vi "Process_Setting_UI2.vi"(9 "Image In":T2, 10 "PreProcess":T1=enum."G_Threshold", 11 "DataIn":string) -> (1 "ExitFLG":bool=TRUE, 3 "DataOut":string)   [LabVIEW 2019]
uses:
  Controls/MaskParam_Type.ctl
  Controls/ParticleFilterParam_Type.ctl
  Controls/LookupTableParam.ctl
  Controls/FiltersParam_Type.ctl
  Controls/GrayMorphologyParam_Type.ctl
  Controls/OperatorsParam_Type.ctl
  Controls/BinaryMonoParam_Type.ctl
  Controls/ExtractPlanParam_Type.ctl
  Controls/UI_Process_Type.ctl
  Controls/ProcessBrightness.ctl
  <vilib>/vision/Image Controls.llb/IMAQ Image.ctl
  Ctrl/VisionProcessName.ctl
  Controls/ProcessColorThreshold.ctl
  Controls/Process_Setting.ctl
  30020945-ae28-4489-8016-9b1403305c34.vi
  ebb7c46e-89fc-4514-88ba-51094c50cf0f.vi
  e91a7cad-c41a-4cff-b925-06470bbe3936.vi
  b75ec72d-941b-4609-8ea7-277ce8708de0.vi
  47af210a-8923-444f-9ea8-79f9655d5eab.vi
  a8380952-e245-4862-98bc-7050634aa2b9.vi
  c91c66e3-d08b-4d8f-9520-13536894a5b1.vi
  b6b5b608-5e76-4822-9d65-04a57b09488a.vi
  97fa0709-478f-42d9-9b21-5a1c8d8fbb1e.vi
  9fa7adbb-d216-4a6e-bf6a-ec4f0884b3b2.vi
  99202b2e-11d4-433c-aa93-4f5d47ce0152.vi
  de4bf947-11f1-4644-b15e-f20b2debb1f4.vi
  d1f0ac64-7591-4813-b16e-cc2f2336aeb7.vi
  21e68b17-46f9-4e60-a793-2575703a9335.vi
  2b11d1c0-0739-46ad-be8a-3e73a10ae897.vi
  6a6545d9-b3d5-4342-817e-e9b56ae9a0c9.vi
  33d971b2-c2c9-4da8-8c72-03e55e502448.vi
  e97b490d-7b27-4472-b442-b6ae32428c3c.vi
  <vilib>/JDP Science/JSONtext/Variant to JSON Text.vi
  <vilib>/JDP Science/JSONtext/JSON text to Variant.vi
  ccb8fe9b-0148-4a2a-9ee9-959eed898db8.vi
  76e84c50-6107-4eeb-8902-48fd924c973a.vi
  068fea54-6e28-4c40-a19e-0b6ebeaa2479.vi
  293cadd9-7c19-42b2-90f6-8eb66fc12dc6.vi
  ad7b33dd-2a70-464f-aced-769d5ac39227.vi
panel:
  in  "ParticleFilterParam":T3={"Selection Values"=[], "Keep/Remove Particles (F)"=FALSE, "Reject Border? (F)"=FALSE, "Fill Holes? (F)"=FALSE, "Connectivity 4/8 (8)"=TRUE} {"Selection Values"."Measurement Parameter" items=["Center of Mass X", "Center of Mass Y", "First Pixel X", "First Pixel Y", "Bounding Rect Left", "Bounding Rect Top", "Bounding Rect Right", "Bounding Rect Bottom", "Max Feret Diameter Start X", "Max Feret Diameter Start Y", "Max Feret Diameter End X", "Max Feret Diameter End Y", "Max Horiz. Segment Length Left", "Max Horiz. Segment Length Right", "Max Horiz. Segment Length Row", "-", "Bounding Rect Width", "Bounding Rect Height", "Bounding Rect Diagonal", "Perimeter", "Convex Hull Perimeter", "Holes' Perimeter", "Max Feret Diameter", "Equivalent Ellipse Major Axis", "Equivalent Ellipse Minor Axis", "Equivalent Ellipse Minor Axis (Feret)", "Equivalent Rect Long Side", "Equivalent Rect Short Side", "Equivalent Rect Diagonal", "Equivalent Rect Short Side (Feret)", "Average Horiz. Segment Length", "Average Vert. Segment Length", "Hydraulic Radius", "Waddel Disk Diameter", "-", "Area", "Holes' Area", "Particle & Holes' Area", "Convex Hull Area", "Image Area", "-", "Number of Holes", "Number of Horiz. Segments", "Number of Vert. Segments", "-", "Orientation", "Max Feret Diameter Orientation", "-", "% Area/Image Area", "% Area/(Particle & Holes' Area)", "Ratio of Equivalent Ellipse Axes", "Ratio of Equivalent Rect Sides", "-", "Elongation Factor", "Compactness Factor", "Heywood Circularity Factor", "Type Factor", "-", "Sum X", "Sum Y", "Sum XX", "Sum XY", "Sum YY", "Sum XXX", "Sum XXY", "Sum XYY", "Sum YYY", "-", "Moment of Inertia XX", "Moment of Inertia XY", "Moment of Inertia YY", "Moment of Inertia XXX", "Moment of Inertia XXY", "Moment of Inertia XYY", "Moment of Inertia YYY", "Norm. Moment of Inertia XX", "Norm. Moment of Inertia XY", "Norm. Moment of Inertia YY", "Norm. Moment of Inertia XXX", "Norm. Moment of Inertia XXY", "Norm. Moment of Inertia XYY", "Norm. Moment of Inertia YYY", "Hu Moment 1", "Hu Moment 2", "Hu Moment 3", "Hu Moment 4", "Hu Moment 5", "Hu Moment 6", "Hu Moment 7"]; "Selection Values"."Range Lower Value" format="%.2f"; "Selection Values"."Range Upper Value" format="%.2f"}
  in  "GrayMorphologyParam":T5={"Operation"=enum."AutoM", "Structuring Element"=[[1, 1, 1], [1, 1, 1], [1, 1, 1]], "Square/Hexa (Square)"=FALSE, "Number of iterations"=1}
  in  "OperatorsParam":T6
  out "Operators_Image":T2(plugin-control)
  in  "Tab Control":enum32{"Page 1", "Page 2"}(tab)
  in  "Btn_Cancel":bool
  in  "Btn_Set":bool
  out "Image":T2(plugin-control)
  in  "Tab":T7=enum."ExtractPlane"
  in  "Brightness":T8={"Brightness"=0, "Constrast"=1.0, "Gamma"=0.0} {"Gamma" scale=10.0..0.1 scale format="%#_1f"; "Constrast" min=1.0 max=89.0 scale=1.0..89.0 scale format="%.2f"; "Brightness" min=0 max=255 step=1 scale=0.0..255.0}
  in  "ExtractPlanParam":T9={"Color Plane"=enum."Green"}
  in  "ColorThreshold":T10={"Color Mode"=0, "Red or Hue Range"={120.0, 255.0}, "Green or Sat Range"={120.0, 255.0}, "Blue or Luma or Val or Inten Range"={120.0, 255.0}} {"Blue or Luma or Val or Inten Range" scale=0.0..255.0; "Green or Sat Range" scale=0.0..255.0; "Red or Hue Range" scale=0.0..255.0; "Color Mode" items=["RGB", "HSL", "HSV", "HSI"]}
  in  "LookupTableParam":T11={"Function"=enum."Power X", "Power Value"=1.5}
  in  "FiltersParam":T12={"Kernel"=[[1.0, 1.0, 1.0], [1.0, 1.0, 1.0], [1.0, 1.0, 1.0]], "Kernel Size"=0, "Filter Size X"=0, "Filter Size Y"=0, "Tolerance %"=0, "Divider"=0.0, "FilterFunction"=enum."Smoothing - Low Pass", "Sigma"=0.0, "LThres"=0.0, "HThresh"=0.0, "Windows Size"=0} {"Kernel Size" min=3 max=7 step=2}
  in  "MonoThreshold":T13={"Look For"=enum."Bright Objects", "Threshold"={120.0, 255.0}} {"Threshold" scale=0.0..255.0}
  in  "MaskParam":T14
  # "Minimum"
  # "Maximum"
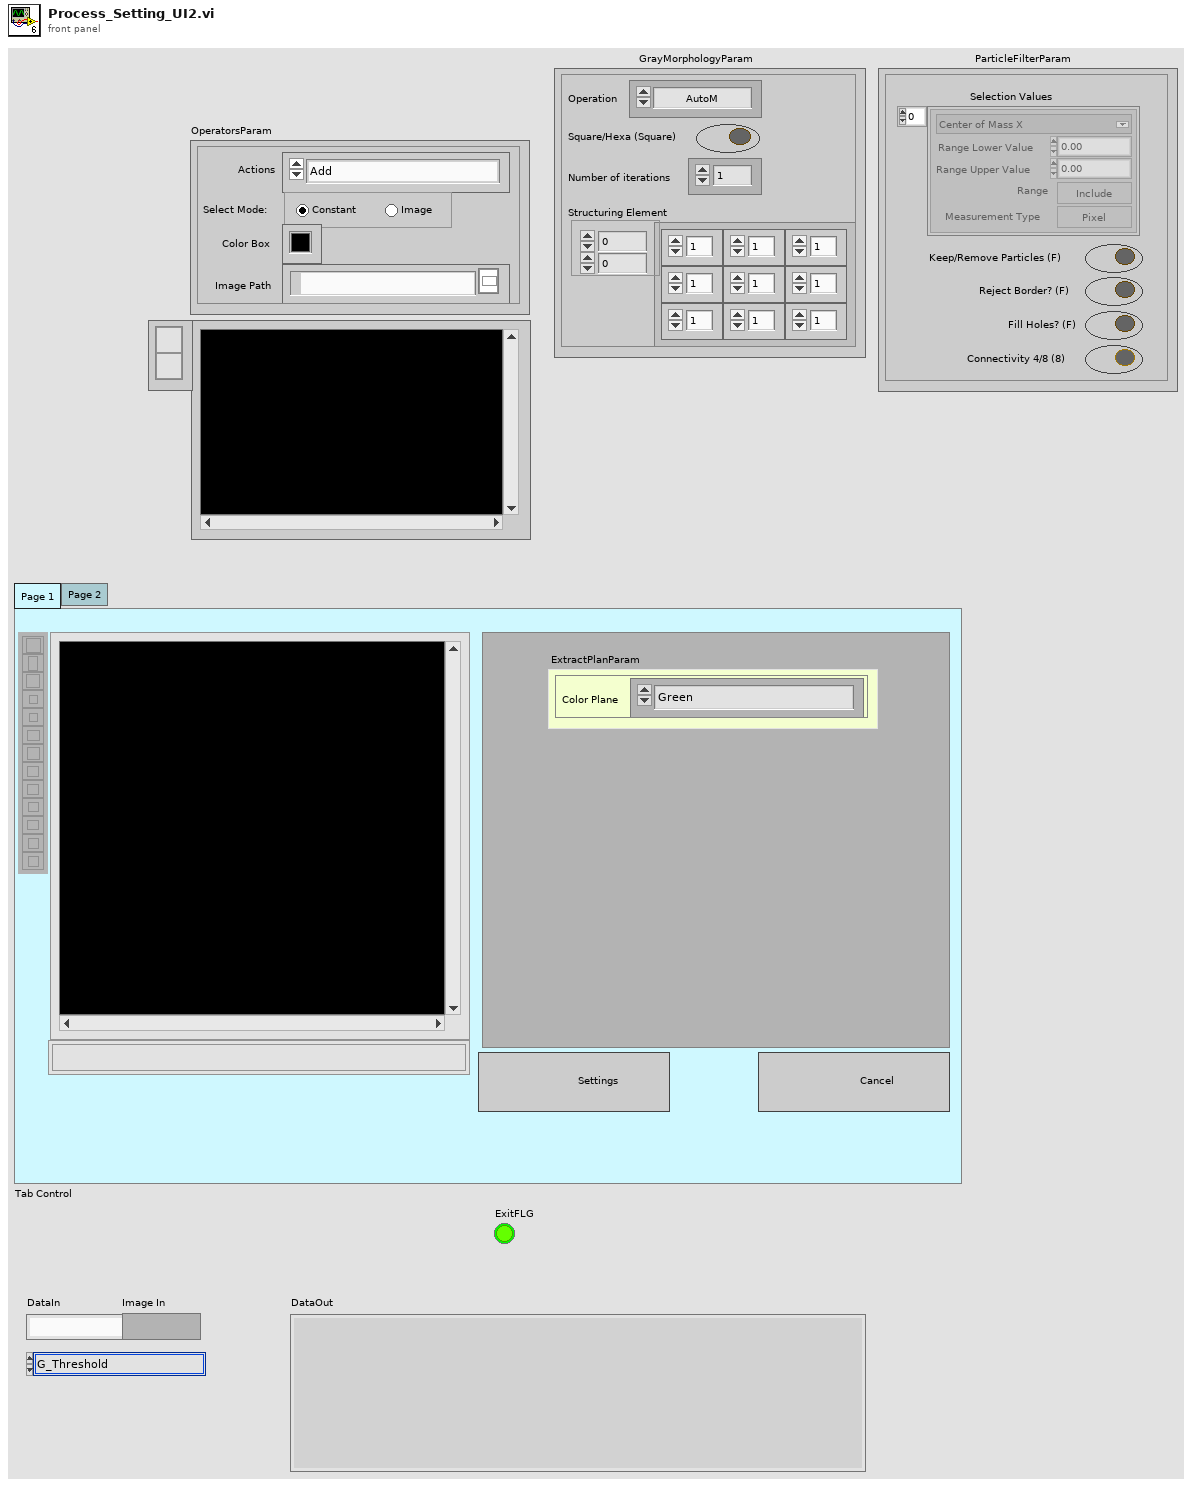
[diagram p1: front panel]
types:
  T1 = typedef "VisionProcessName.ctl" = enum16{"*CamParameter*", "CamAttributes", "*Preprocess*", "CG_Brightness", "C_Plane Extraction", "C_Threshold", "G_Lookup Table", "G_Threshold"}
  T2 = typedef "IMAQ Image.ctl" = refnum<image>
  T3 = typedef "ParticleFilterParam_Type.ctl" = cluster{"Selection Values":cluster{"Measurement Parameter":T4, "Range Lower Value":dbl, "Range Upper Value":dbl, "Range":bool, "Measurement Type":bool}[], "Keep/Remove Particles (F)":bool, "Reject Border? (F)":bool, "Fill Holes? (F)":bool, "Connectivity 4/8 (8)":bool}
  T4 = typedef "Particle Parameters" = i32
  T5 = typedef "GrayMorphologyParam_Type.ctl" = cluster{"Operation":enum32{"AutoM", "Close", "Dilate", "Erode", "Gradient", "Gradient in", "Gradient out", "HitMiss", "Open", "PClose", "POpen", "Thick", "Thin"}, "Structuring Element":i32[][], "Square/Hexa (Square)":bool, "Number of iterations":i32}
  T6 = typedef "OperatorsParam_Type.ctl" = cluster{"Actions":enum16{"Add", "Subtract", "Multiply", "Divide", "Multiply Divide", "Modulo", "Absolutio Difference", "---------------------------------", "And", "Not And", "Or", "Not Or", "Exclusive Or", "Not Exclusive Or", "Logical Difference", "----------------------------------", "Mask"}, "Select Mode:":enum32{"Constant", "Image"}, "Color Box":u32, "Image Path":path}
  T7 = typedef "UI_Process_Type.ctl" = enum32{"None", "Brightness", "ExtractPlane", "CThreshold", "Lookup Table", "Filters", "GrayMorphology", "GThreshold", "Operators", "Particle Filter", "Mask"}
  T8 = typedef "ProcessBrightness.ctl" = cluster{"Brightness":i32, "Constrast":dbl, "Gamma":dbl}
  T9 = typedef "ExtractPlanParam_Type.ctl" = cluster{"Color Plane":enum16{"Red", "Green", "Blue", "Hue", "Saturation", "Luminance", "Value", "Intensity"}}
  T10 = typedef "ProcessColorThreshold.ctl" = cluster{"Color Mode":u16, "Red or Hue Range":cluster{dbl, dbl}, "Green or Sat Range":cluster{dbl, dbl}, "Blue or Luma or Val or Inten Range":cluster{dbl, dbl}}
  T11 = typedef "LookupTableParam.ctl" = cluster{"Function":enum16{"Equalizer", "Reverse", "Logarithmic", "Exponential", "Square", "Square Root", "Power X", "Power 1/X"}, "Power Value":sgl}
  T12 = typedef "FiltersParam_Type.ctl" = cluster{"Kernel":sgl[][], "Kernel Size":i32, "Filter Size X":i32, "Filter Size Y":i32, "Tolerance %":i32, "Divider":sgl, "FilterFunction":enum16{"Smoothing - Low Pass", "Smoothing - Local Average", "Smoothing - Guassian", "Smoothing - Median", "------------------------------------", "Edge Detection - Laplacian", "Edge Detection - Diff", "Edge Detection - Prewitt", "Edge Detection - Sobel", "Edge Detection - Roberts", "Edge Detection - Canny", "Edge Detection - Gradient", "Edge Detection - Sigma", "----------------------------------------", "Convolution - Highlight Details", "Convolution - Custom"}, "Sigma":sgl, "LThres":sgl, "HThresh":sgl, "Windows Size":i32}
  T13 = typedef "BinaryMonoParam_Type.ctl" = cluster{"Look For":enum16{"Bright Objects", "Dark Objects", "Gray Objects"}, "Threshold":cluster{dbl, dbl}}
  T14 = typedef "MaskParam_Type.ctl" = cluster{"Function":enum16{"Inside", "Outside"}, "ROI List":i32, "ROI":cluster{"Global Rectangle":i32[], "Contours":cluster{"Contour Type":u32, "ROI Type":u32, "Points":i32[]}[]}[], "Creat ROI":bool, "Delete ROI":bool, "Enabled/Disabled":bool, "Color Box":u32, "Last Mouse Position":cluster{"X":i32, "Y":i32}}
  T15 = typedef "Process_Setting.ctl" = cluster{"Enum_PreProcess":T1, "Parameter":string}
  T16 = typedef "Image Type" = u32
  T17 = enum16{"Bright Objects", "Dark Objects", "Gray Objects"}
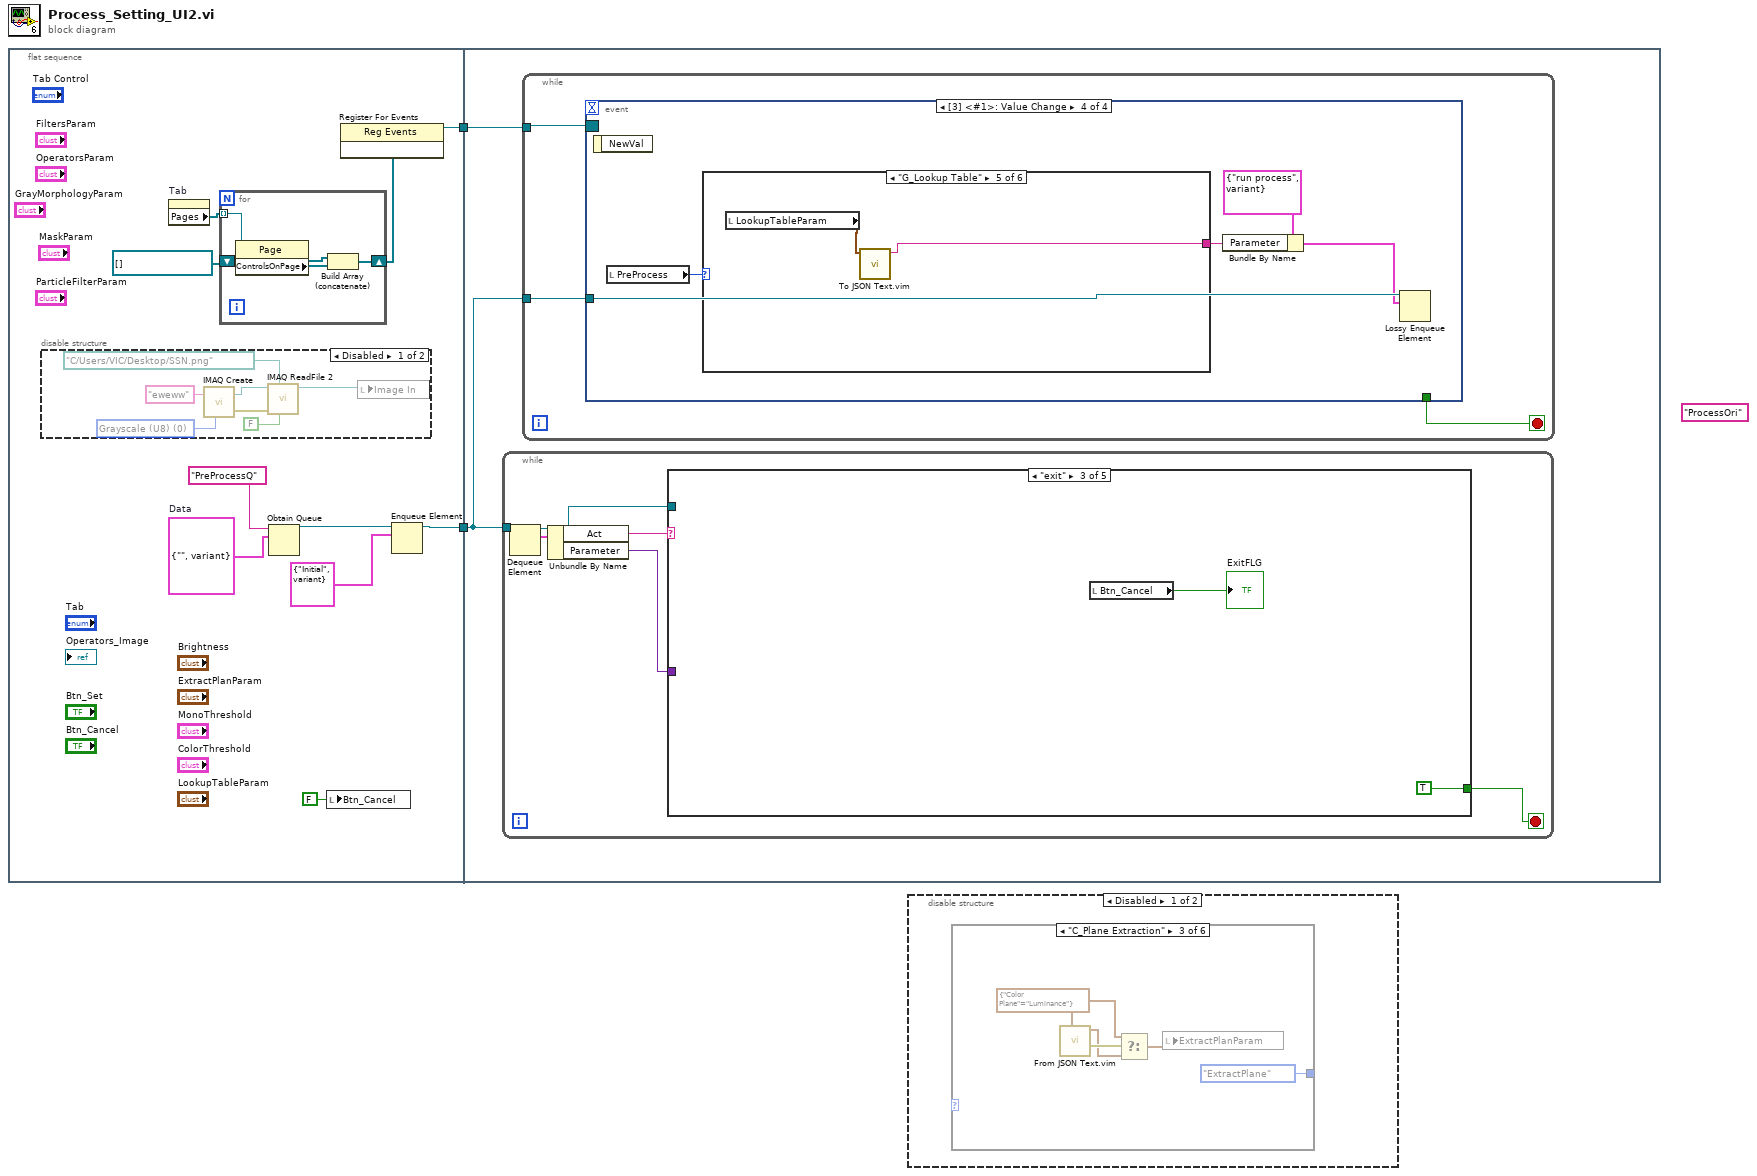
[diagram p0: block diagram]
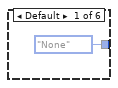
[diagram p2: hidden frame]
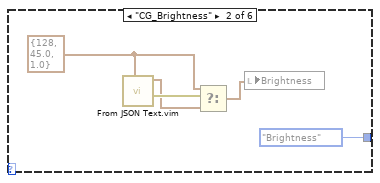
[diagram p3: hidden frame]
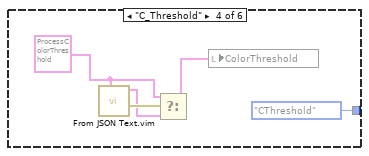
[diagram p4: hidden frame]
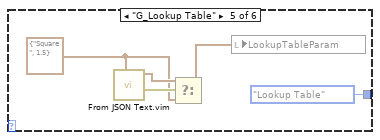
[diagram p5: hidden frame]
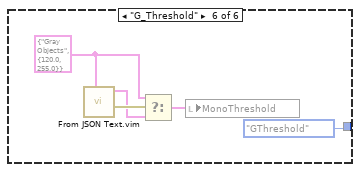
[diagram p6: hidden frame]
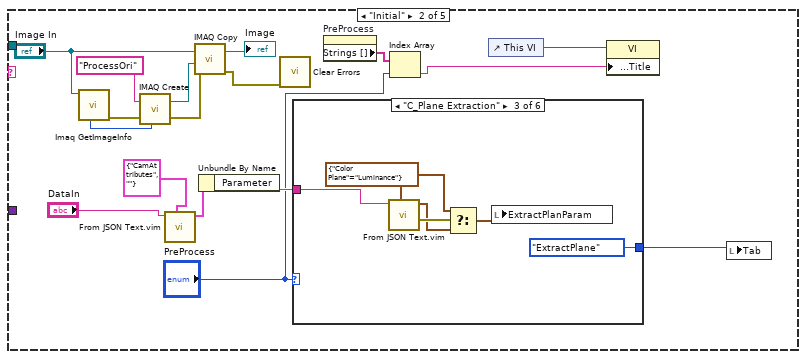
[diagram p10: hidden frame]
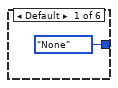
[diagram p11: hidden frame]
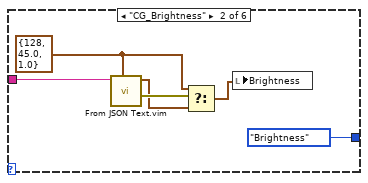
[diagram p12: hidden frame]
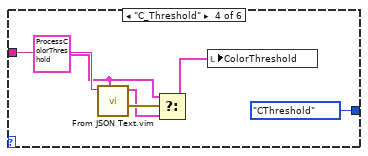
[diagram p13: hidden frame]
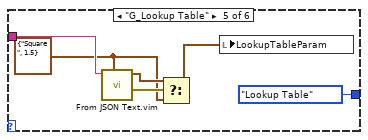
[diagram p14: hidden frame]
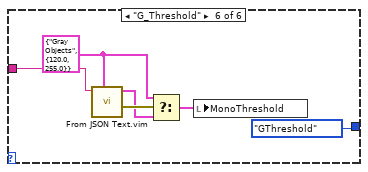
[diagram p15: hidden frame]
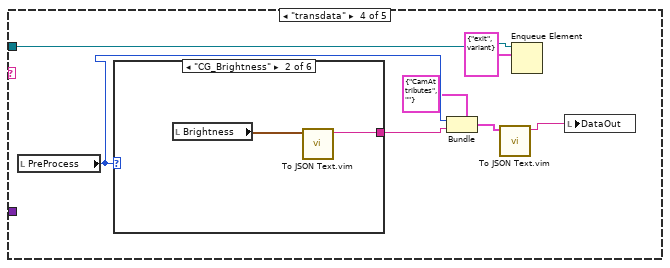
[diagram p16: hidden frame]
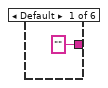
[diagram p17: hidden frame]
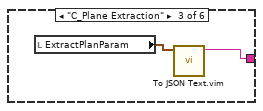
[diagram p18: hidden frame]
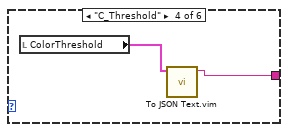
[diagram p19: hidden frame]
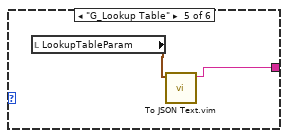
[diagram p20: hidden frame]
diagram:
  (unwired) "ProcessOri" ("Image Name")
  n1 = flat-sequence {
    tunnel: [w9] -> w2
    tunnel: [w7] -> w1
    tunnel: w2 -> [w25]
    tunnel: w1 -> [w24]
    frame #0 {
      w11 = cluster{"Act":string, "Parameter":variant} {"Act"="", "Parameter"=variant}  # Data
      n2 = disable-structure shown="Disabled" {
        frame Disabled {
          w14 = T16 0 items=["Grayscale (U8)", "Grayscale (I16)", "Grayscale (SGL)", "Complex (CSG)", "RGB (U32)", "HSL (U32)", "RGB (U64)", "Grayscale (U16)"] ("Image Type")
          n3 = call "IMAQ Create"("Image Name"="eweww", "Image Type"=w14) -> ("New Image"=w15:T2, "error out"=w16:errorcluster)  [unwired: 3 in]
          n4 = call "IMAQ ReadFile 2"("Use File Path Image Type"=FALSE, "File Path"=path "C:/Users/VIC/Desktop/SSN.png", "error in (no error)"=w16, "Image"=w15) -> ("Image Out"=w18:T2)  [unwired: 3 in, 4 out]
          n5 = local write "Image In"(w18) -> ()
        }
        frame Enabled {
        }
      }
      n6 = property on="Tab" class="TabCtl (strict)"() -> ("Pages"=w6:refnum<vi>[])  [unwired: 2 in, 2 out]
      n7 = for {
        tunnel: w6 -> [w23] mode=indexing
        shift-right: [w21] -> w4
        shift-left: refnum<vi>[] [] -> [w20]
        n8 = property class="Page"(reference=w23) -> ("ControlsOnPage"=w22:refnum<vi>[])  [unwired: 1 in, 2 out]
        n9 = Build Array (concatenate)(w20, w22) -> (w21:refnum<vi>[])
      }
      n10 = Obtain Queue(name (unnamed)="PreProcessQ", element data type=w11) -> (queue out=w10:refnum<queue>)  [unwired: 3 in, 2 out]
      n11 = local write "Btn_Cancel"(FALSE ("Btn_Cancel")) -> ()
      n12 = register-events(w4) -> (reference out=w7:refnum<event-registration>)  [unwired: 2 in, 1 out]
      n13 = Enqueue Element(queue=w10, element=cluster{"Act":string, "Parameter":variant} {"Act"="Initial", "Parameter"=variant}) -> (queue out=w9:refnum<queue>)  [unwired: 2 in, 2 out]
    }
    frame #1 {
      n14 = while {
        tunnel: w25 -> [w31]
        stop <- w28 stop-if-true
        n15 = Dequeue Element(queue=w31) -> (queue out=w27:refnum<queue>, element=w30:cluster{"Act":string, "Parameter":variant})  [unwired: 2 in, 2 out]
        n16 = Unbundle By Name(w30) -> ("Act"=w29:string, "Parameter"=w26:variant)
        n17 = case shown="\"exit\"" w29 {
          tunnel: [_ _ TRUE _ _] -> w28
          tunnel: w27 -> [_ _ _ w88 _]
          tunnel: w26 -> [_ _ _ _ w107]
          frame "False", Default {
          }
          frame "Initial" {
            n18 = call "Imaq GetImageInfo"("Image"="Image In") -> ("error out"=w44:errorcluster, "Image Type"=w47:T16)  [unwired: 3 in, 6 out]
            n19 = call "IMAQ Create"("Image Name"="ProcessOri", "Image Type"=w47, "error in (no error)"=w44) -> ("New Image"=w45:T2, "error out"=w43:errorcluster)  [unwired: 2 in]
            n20 = call "From JSON Text.vim"("Data Type and Default Value"=T15 {"Enum_PreProcess"=enum."CamAttributes", "Parameter"=""} ("ProcessSetting"), "JSON"="DataIn") -> ("Data out"=w37:T15)  [unwired: 8 in, 1 out]
            n21 = call "IMAQ Copy"("error in (no error)"=w43, "Image Dst"=w45, "Image Src"="Image In") -> ("error out"=w40:errorcluster, "Image Dst Out"=→"Image":T2)  [unwired: 3 in]
            n22 = Unbundle By Name(w37) -> ("Parameter"=w38:string)
            n23 = call <vilib>:"Clear Errors.vi"("error in (no error)"=w40) -> ()  [unwired: 5 in, 2 out]
            n24 = case shown="\"C_Plane Extraction\"" "PreProcess" {
              tunnel: w38 -> [_ w55 w61 w66 w72 w78]
              tunnel: [UI_Process_Type."None" ("Tab") UI_Process_Type."Brightness" ("Tab") UI_Process_Type."ExtractPlane" ("Tab") UI_Process_Type."CThreshold" ("Tab") UI_Process_Type."Lookup Table" ("Tab") UI_Process_Type."GThreshold" ("Tab")] -> w41
              frame Default {
              }
              frame "CG_Brightness" {
                w51 = T8 {"Brightness"=128, "Constrast"=45.0, "Gamma"=1.0} ("t")
                n25 = call "From JSON Text.vim"("Data Type and Default Value"=w51, "JSON"=w55) -> ("error out"=w54:errorcluster, "Data out"=w52:T8)  [unwired: 8 in]
                n26 = Select(t=w51, s=w54, f=w52) -> (s? t:f=w53:T8)
                n27 = local write "Brightness"(w53) -> ()
              }
              frame "C_Plane Extraction" {
                w57 = T9 {"Color Plane"=enum."Luminance"} ("ExtractPlanParam")
                n28 = call "From JSON Text.vim"("Data Type and Default Value"=w57, "JSON"=w61) -> ("error out"=w60:errorcluster, "Data out"=w59:T9)  [unwired: 8 in]
                n29 = Select(t=w57, s=w60, f=w59) -> (s? t:f=w58:T9)
                n30 = local write "ExtractPlanParam"(w58) -> ()
              }
              frame "C_Threshold" {
                w65 = T10 {"Color Mode"=0, "Red or Hue Range"={120.0, 255.0}, "Green or Sat Range"={120.0, 255.0}, "Blue or Luma or Val or Inten Range"={120.0, 255.0}} ("ColorThreshold")
                n31 = call "From JSON Text.vim"("Data Type and Default Value"=w65, "JSON"=w66) -> ("error out"=w67:errorcluster, "Data out"=w63:T10)  [unwired: 8 in]
                n32 = Select(t=w65, s=w67, f=w63) -> (s? t:f=w64:T10)
                n33 = local write "ColorThreshold"(w64) -> ()
              }
              frame "G_Lookup Table" {
                w70 = T11 {"Function"=enum."Square", "Power Value"=1.5} ("LookupTableParam")
                n34 = call "From JSON Text.vim"("Data Type and Default Value"=w70, "JSON"=w72) -> ("error out"=w73:errorcluster, "Data out"=w71:T11)  [unwired: 8 in]
                n35 = Select(t=w71, s=w73, f=w70) -> (s? t:f=w69:T11)
                n36 = local write "LookupTableParam"(w69) -> ()
              }
              frame "G_Threshold" {
                w76 = T13 {"Look For"=enum."Gray Objects", "Threshold"={120.0, 255.0}} ("MonoThreshold")
                n37 = call "From JSON Text.vim"("Data Type and Default Value"=w76, "JSON"=w78) -> ("error out"=w79:errorcluster, "Data out"=w77:T13)  [unwired: 8 in]
                n38 = Select(t=w76, s=w79, f=w77) -> (s? t:f=w75:T13)
                n39 = local write "MonoThreshold"(w75) -> ()
              }
            }
            n40 = property on="PreProcess" class="Enum (strict)"() -> ("Strings []"=w34:string[])  [unwired: 2 in, 2 out]
            n41 = Index Array(array=w34, index="PreProcess") -> (element=w32:string)
            n42 = control-ref of="This VI"() -> (w35:refnum<vi>)
            n43 = property class="VI"(reference=w35, "Front Panel.Title"=w32) -> ()  [unwired: 1 in, 2 out]
            n44 = local write "Tab"(w41) -> ()
          }
          frame "exit" {
            n45 = local read "Btn_Cancel"() -> (→"ExitFLG":bool)
          }
          frame "transdata" {
            n46 = local read "PreProcess"() -> (w83:T1)
            n47 = case shown="\"CG_Brightness\"" w83 {
              tunnel: ["" ("<JSON>") w90 w93 w94 w96 w98] -> w86
              frame Default {
              }
              frame "CG_Brightness" {
                n48 = local read "Brightness"() -> (w91:T8)
                n49 = call "To JSON Text.vim"("Anything"=w91) -> ("<JSON>"=w90:string)  [unwired: 9 in, 1 out]
              }
              frame "C_Plane Extraction" {
                n50 = local read "ExtractPlanParam"() -> (w92:T9)
                n51 = call "To JSON Text.vim"("Anything"=w92) -> ("<JSON>"=w93:string)  [unwired: 9 in, 1 out]
              }
              frame "C_Threshold" {
                n52 = local read "ColorThreshold"() -> (w95:T10)
                n53 = call "To JSON Text.vim"("Anything"=w95) -> ("<JSON>"=w94:string)  [unwired: 9 in, 1 out]
              }
              frame "G_Lookup Table" {
                n54 = local read "LookupTableParam"() -> (w97:T11)
                n55 = call "To JSON Text.vim"("Anything"=w97) -> ("<JSON>"=w96:string)  [unwired: 9 in, 1 out]
              }
              frame "G_Threshold" {
                n56 = local read "MonoThreshold"() -> (w99:T13)
                n57 = call "To JSON Text.vim"("Anything"=w99) -> ("<JSON>"=w98:string)  [unwired: 9 in, 1 out]
              }
            }
            n58 = Bundle(cluster=T15 {"Enum_PreProcess"=enum."CamAttributes", "Parameter"=""} ("ProcessSetting"), "Enum_PreProcess"=w83, "Parameter"=w86) -> (w85:T15)
            n59 = call "To JSON Text.vim"("Anything"=w85) -> ("<JSON>"=w84:string)  [unwired: 9 in, 1 out]
            n60 = Enqueue Element(queue=w88, element=cluster{"Act":string, "Parameter":variant} {"Act"="exit", "Parameter"=variant}) -> ()  [unwired: 2 in, 3 out]
            n61 = local write "DataOut"(w84) -> ()
          }
          frame "run process" {
            w105 = "ProcessOri" ("Image Name")
            n62 = local read "PreProcess"() -> (w100:T1)
            n63 = Variant To Data(type="", Variant=w107) -> (data=w104:string)  [unwired: 1 in, 1 out]
            n64 = call "Imaq GetImageInfo"("Image"=w105) -> ("error out"=w111:errorcluster, "Image Type"=w112:T16)  [unwired: 3 in, 6 out]
            n65 = Bundle(cluster=T15 {"Enum_PreProcess"=enum."CamAttributes", "Parameter"=""} ("ProcessSetting"), "Enum_PreProcess"=w100, "Parameter"=w104) -> (w103:T15)
            n66 = call "To JSON Text.vim"("Anything"=w103) -> ("<JSON>"=w102:string)  [unwired: 9 in, 1 out]
            n67 = call "Preprocess Action.vi"("Image Type"=w112, "Image Dust"="run process" ("Image Name"), "ImageSorce"=w105, "PreProcess"=w100, "error in (no error)"=w111, "Data"=w102) -> ("Refnum out"=w109:T2, "error out"=w108:errorcluster)  [unwired: 8 in]
            n68 = case shown="Error .." w108 {
              selector: w108 -> [_ w115]
              tunnel: w109 -> [w113 _]
              frame No Error {
                n69 = local write "Image"(w113) -> ()
              }
              frame Error {
                n70 = Unbundle By Name(w115) -> ("source"=w114:string)
                n71 = One Button Dialog(message=w114) -> ()  [unwired: 1 in, 1 out]
              }
            }
          }
        }
      }
      n72 = while {
        tunnel: w25 -> [w118]
        tunnel: w24 -> [w116]
        stop <- w117 stop-if-true
        n73 = event shown="[3] <#1>: Value Change" {
          selector: w116 -> [_ _ _ _]
          dyn-events: _ -> [_ _ _ _]
          timeout: _ -> [_ _ _ _]
          tunnel: w118 -> [_ w119 w124 w133]
          tunnel: [_ TRUE TRUE _] -> w117
          event Timeout {
            n74 = event-data() -> ()  [unwired: 1 in, 3 out]
          }
          event "Btn_Set": Value Change {
            n75 = event-data() -> ()  [unwired: 1 in, 6 out]
            n76 = Enqueue Element(queue=w119, element=cluster{"Act":string, "Parameter":variant} {"Act"="transdata", "Parameter"=variant}) -> ()  [unwired: 2 in, 3 out]
          }
          event "Btn_Cancel": Value Change {
            n77 = event-data() -> ()  [unwired: 1 in, 1 out]
            n78 = flat-sequence {
              tunnel: w124 -> [w126]
              tunnel: [w126] -> w122
              tunnel: w122 -> [w128]
              frame #0 {
                n79 = local read "DataIn"() -> (→"DataOut":string)
              }
              frame #1 {
                n80 = Enqueue Element(queue=w128, element=cluster{"Act":string, "Parameter":variant} {"Act"="exit", "Parameter"=variant}) -> ()  [unwired: 2 in, 3 out]
              }
            }
          }
          event Value Change {
            n81 = event-data() -> ()  [unwired: 1 in, 1 out]
            n82 = local read "PreProcess"() -> (w132:T1)
            n83 = case shown="\"G_Lookup Table\"" w132 {
              tunnel: ["" ("<JSON>") w135 w138 w139 w141 w149] -> w130
              frame Default {
              }
              frame "CG_Brightness" {
                n84 = local read "Brightness"() -> (w136:T8)
                n85 = call "To JSON Text.vim"("Anything"=w136) -> ("<JSON>"=w135:string)  [unwired: 9 in, 1 out]
              }
              frame "C_Plane Extraction" {
                n86 = local read "ExtractPlanParam"() -> (w137:T9)
                n87 = call "To JSON Text.vim"("Anything"=w137) -> ("<JSON>"=w138:string)  [unwired: 9 in, 1 out]
              }
              frame "C_Threshold" {
                n88 = local read "ColorThreshold"() -> (w140:T10)
                n89 = call "To JSON Text.vim"("Anything"=w140) -> ("<JSON>"=w139:string)  [unwired: 9 in, 1 out]
              }
              frame "G_Lookup Table" {
                n90 = local read "LookupTableParam"() -> (w142:T11)
                n91 = call "To JSON Text.vim"("Anything"=w142) -> ("<JSON>"=w141:string)  [unwired: 9 in, 1 out]
              }
              frame "G_Threshold" {
                n92 = local read "MonoThreshold"() -> (w146:T13)
                n93 = Unbundle(w146) -> ("Look For"=w147:T17, "Threshold"=w148:cluster{dbl, dbl})
                n94 = Unbundle(w148) -> (w144:dbl, w145:dbl)
                n95 = case shown="\"Gray Objects\", Default" w147 {
                  tunnel: w146 -> [w150 w159 w160]
                  tunnel: [w153 w158 w160] -> w143
                  tunnel: w145 -> [_ w156 _]
                  tunnel: w144 -> [w152 _ _]
                  frame "Bright Objects" {
                    n96 = Bundle(w152, 255.0) -> (w154:cluster{dbl, dbl})  [unwired: 1 in]
                    n97 = Bundle By Name(cluster=w150, "Threshold"=w154) -> (w153:T13)
                  }
                  frame "Dark Objects" {
                    n98 = Bundle(0.0, w156) -> (w157:cluster{dbl, dbl})  [unwired: 1 in]
                    n99 = Bundle By Name(cluster=w159, "Threshold"=w157) -> (w158:T13)
                  }
                  frame "Gray Objects", Default {
                  }
                }
                n100 = local write "MonoThreshold"(w143) -> ()
                n101 = call "To JSON Text.vim"("Anything"=w143) -> ("<JSON>"=w149:string)  [unwired: 9 in, 1 out]
              }
            }
            n102 = Bundle By Name(cluster=cluster{"Act":string, "Parameter":variant} {"Act"="run process", "Parameter"=variant} ("element"), "Parameter"=w130) -> (w129:cluster{"Act":string, "Parameter":variant})
            n103 = Lossy Enqueue Element(queue=w133, element=w129) -> ()  [unwired: 1 in, 4 out]
          }
        }
      }
    }
  }
  n104 = disable-structure shown="Disabled" {
    frame Disabled {
      n105 = case shown="\"C_Plane Extraction\"" {
        selector: _ -> [_ _ _ _ _ _]
        tunnel: [UI_Process_Type."None" ("Tab") UI_Process_Type."Brightness" ("Tab") UI_Process_Type."ExtractPlane" ("Tab") UI_Process_Type."CThreshold" ("Tab") UI_Process_Type."Lookup Table" ("Tab") UI_Process_Type."GThreshold" ("Tab")] -> _
        frame Default {
        }
        frame "CG_Brightness" {
          w163 = T8 {"Brightness"=128, "Constrast"=45.0, "Gamma"=1.0} ("t")
          n106 = call "From JSON Text.vim"("Data Type and Default Value"=w163) -> ("error out"=w166:errorcluster, "Data out"=w164:T8)  [unwired: 9 in]
          n107 = Select(t=w163, s=w166, f=w164) -> (s? t:f=w165:T8)
          n108 = local write "Brightness"(w165) -> ()
        }
        frame "C_Plane Extraction" {
          w168 = T9 {"Color Plane"=enum."Luminance"} ("ExtractPlanParam")
          n109 = call "From JSON Text.vim"("Data Type and Default Value"=w168) -> ("error out"=w171:errorcluster, "Data out"=w170:T9)  [unwired: 9 in]
          n110 = Select(t=w168, s=w171, f=w170) -> (s? t:f=w169:T9)
          n111 = local write "ExtractPlanParam"(w169) -> ()
        }
        frame "C_Threshold" {
          w175 = T10 {"Color Mode"=0, "Red or Hue Range"={120.0, 255.0}, "Green or Sat Range"={120.0, 255.0}, "Blue or Luma or Val or Inten Range"={120.0, 255.0}} ("ColorThreshold")
          n112 = call "From JSON Text.vim"("Data Type and Default Value"=w175) -> ("error out"=w176:errorcluster, "Data out"=w173:T10)  [unwired: 9 in]
          n113 = Select(t=w175, s=w176, f=w173) -> (s? t:f=w174:T10)
          n114 = local write "ColorThreshold"(w174) -> ()
        }
        frame "G_Lookup Table" {
          w179 = T11 {"Function"=enum."Square", "Power Value"=1.5} ("LookupTableParam")
          n115 = call "From JSON Text.vim"("Data Type and Default Value"=w179) -> ("error out"=w181:errorcluster, "Data out"=w180:T11)  [unwired: 9 in]
          n116 = Select(t=w180, s=w181, f=w179) -> (s? t:f=w178:T11)
          n117 = local write "LookupTableParam"(w178) -> ()
        }
        frame "G_Threshold" {
          w184 = T13 {"Look For"=enum."Gray Objects", "Threshold"={120.0, 255.0}} ("MonoThreshold")
          n118 = call "From JSON Text.vim"("Data Type and Default Value"=w184) -> ("error out"=w186:errorcluster, "Data out"=w185:T13)  [unwired: 9 in]
          n119 = Select(t=w184, s=w186, f=w185) -> (s? t:f=w183:T13)
          n120 = local write "MonoThreshold"(w183) -> ()
        }
      }
    }
    frame Enabled {
    }
  }
